vi "Read Single.vi"() -> ()   [LabVIEW 2013]
doc: "This example shows how to configure a measurement and take a reading."
uses:
  <instrlib>/Keithley 24XX/Public/Data/Read (Single Point).vi
  <vilib>/Utility/file.llb/Read From Spreadsheet File (DBL).vi
  <instrlib>/Keithley 24XX/Keithley 24XX.lvlib
  <vilib>/gmath/NI_Gmath.lvlib
panel:
  out "Temperature":dbl
  in  "定标文件":string(combo)
  in  "Source Mode  (0: Voltage)":u16(ring) items=["Voltage", "Current"]
  in  "Compliance  Level (0.1)":dbl=0.1
  in  "Output Level (0)":dbl
  in  "Enable Resistance Auto Range (T:Enable)":bool=TRUE
  in  "Enable Current Auto Range (T:Enable)":bool=TRUE
  in  "Enable Voltage Auto Range (T:Enable)":bool=TRUE
  in  "Resistance Manual Range (1.0)":dbl=1.0
  in  "Current Manual Range (1.0)":dbl=1.0
  in  "Voltage Manual Range (1.0)":dbl=1.0
  out "Resistance":sgl
  out "Current":sgl
  out "Voltage":sgl
  in  "Serial Configuration":T1={"Baud Rate"=9600, "Parity"=0, "Data Bits"=8, "Stop Bits"=10, "Flow Control"=0} {"Flow Control" items=["None", "XON/XOFF", "RTS/CTS", "XON/XOFF & RTS/CTS", "DTR/DSR", "XON/XOFF & DTR/DSR"]; "Stop Bits" items=["1.0"=10, "1.5"=15, "2.0"=20]; "Data Bits" items=["7"=7, "8"=8]; "Parity" items=["None", "Odd", "Even", "Mark", "Space"]; "Baud Rate" items=["300"=300, "600"=600, "1200"=1200, "2400"=2400, "4800"=4800, "9600"=9600, "19200"=19200]}
  in  "VISA resource name":refnum<visa-resource-name>
  # "Voltage Range Settings"
  # "Current Range Settings"
  # "Resistance Range Settings"
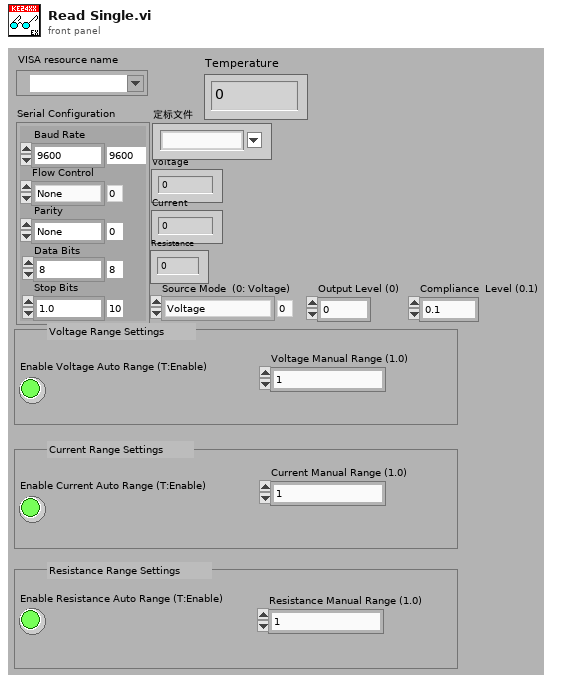
[diagram p1: front panel]
types:
  T1 = cluster{"Baud Rate":u32, "Parity":u16, "Data Bits":u16, "Stop Bits":u16, "Flow Control":u16}
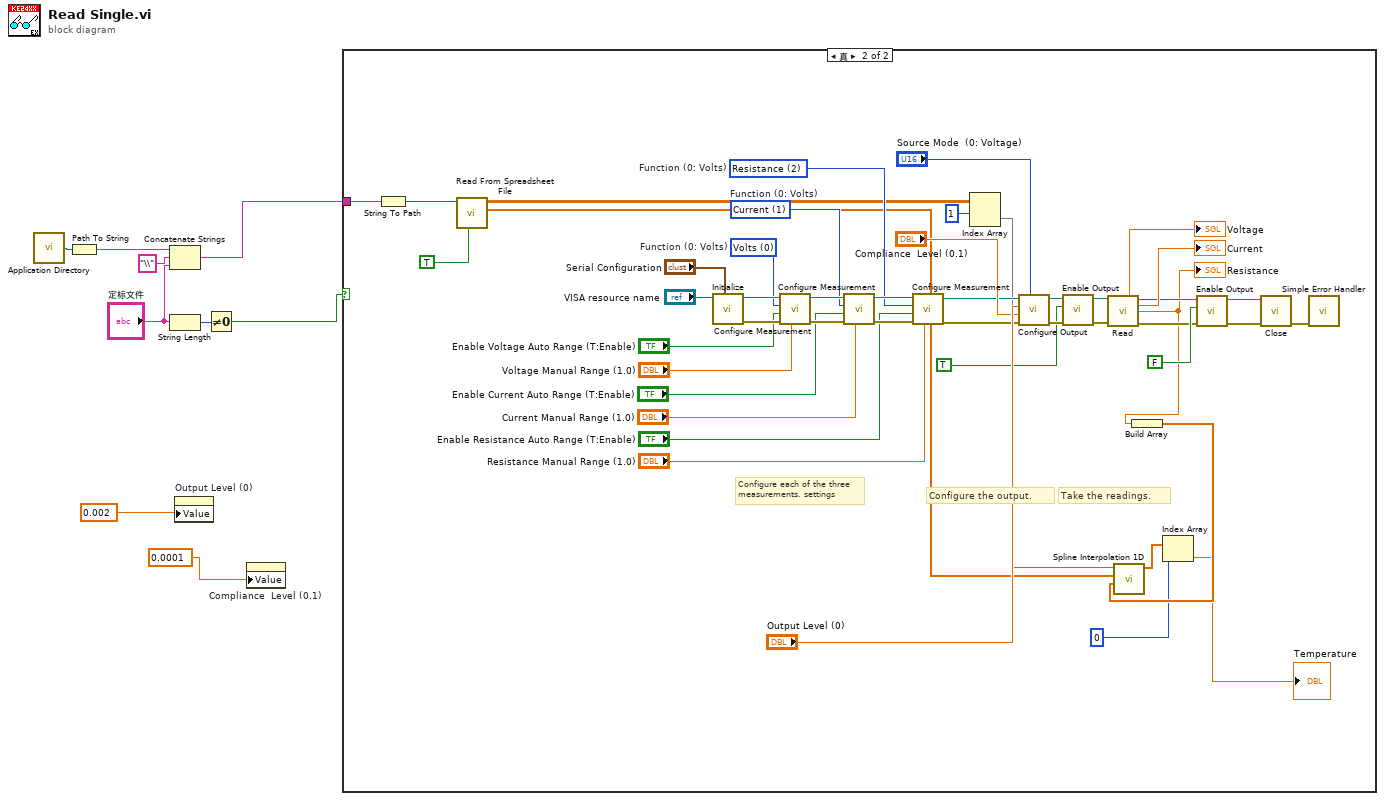
[diagram p0: block diagram]
diagram:
  n1 = call <vilib>:"Application Directory.vi"() -> ("Application Directory"=w9:path)
  n2 = Path To String(path=w9) -> (string=w8:string)
  n3 = Concatenate Strings(w8, "\\", "定标文件") -> (w3:string)
  n4 = String Length(string="定标文件") -> (length=w5:i32)
  n5 = property on="Output Level (0)" class="DigNum (严格)"("Value"=0.002) -> ()  [unwired: 2 in, 2 out]
  n6 = Not Equal To 0?(x=w5) -> (x != 0?=w4:bool)
  n7 = property on="Compliance  Level (0.1)" class="DigNum (严格)"("Value"=0.0001) -> ()  [unwired: 2 in, 2 out]
  n8 = case shown="真" w4 {
    tunnel: w3 -> [_ w16]
    frame False {
    }
    frame True {
      w43 = u16 2 items=["Volts", "Current", "Resistance"]  # Function (0: Volts)
      w44 = u16 1 items=["Volts", "Current", "Resistance"]  # Function (0: Volts)
      w45 = u16 0 items=["Volts", "Current", "Resistance"]  # Function (0: Volts)
      # "Take the readings."
      # "Configure the output."
      # "Configure each of the three measurements. settings"
      n9 = String To Path(string=w16) -> (path=w21:path)
      n10 = call-poly <vilib>:"Read From Spreadsheet File.vi"("transpose (no:F)"=TRUE, "file path (dialog if empty)"=w21) -> ("first row"=w18:dbl[], "all rows"=w19:dbl[][])  [unwired: 5 in, 3 out]
      n11 = call <instrlib>:"Initialize.vi"("Serial Configuration"="Serial Configuration", "VISA resource name"="VISA resource name") -> ("error out"=w50:errorcluster, "VISA resource name out"=w51:refnum<visa-resource-name>)  [unwired: 8 in]
      n12 = call <instrlib>:"Configure Measurement.vi"("Manual Range (1.0)"="Voltage Manual Range (1.0)", "error in (no error)"=w50, "Enable Auto Range (T:Enable)"="Enable Voltage Auto Range (T:Enable)", "Function (0: Volts)"=w45, "VISA resource name"=w51) -> ("error out"=w48:errorcluster, "VISA resource name out"=w49:refnum<visa-resource-name>)  [unwired: 5 in]
      n13 = call <instrlib>:"Configure Measurement.vi"("Manual Range (1.0)"="Current Manual Range (1.0)", "error in (no error)"=w48, "Enable Auto Range (T:Enable)"="Enable Current Auto Range (T:Enable)", "Function (0: Volts)"=w44, "VISA resource name"=w49) -> ("error out"=w47:errorcluster, "VISA resource name out"=w46:refnum<visa-resource-name>)  [unwired: 5 in]
      n14 = call <instrlib>:"Configure Measurement.vi"("Manual Range (1.0)"="Resistance Manual Range (1.0)", "error in (no error)"=w47, "Enable Auto Range (T:Enable)"="Enable Resistance Auto Range (T:Enable)", "Function (0: Volts)"=w43, "VISA resource name"=w46) -> ("error out"=w24:errorcluster, "VISA resource name out"=w23:refnum<visa-resource-name>)  [unwired: 5 in]
      n15 = Index Array(array=w19, index (row)=1) -> (element=w17:dbl[])  [unwired: 1 in]
      n16 = call <instrlib>:"Configure Output.vi"("Source Mode  (0: Voltage)"="Source Mode  (0: Voltage)", "error in (no error)"=w24, "Compliance  Level (0.1)"="Compliance  Level (0.1)", "Output Level (0)"="Output Level (0)", "VISA resource name"=w23) -> ("error out"=w26:errorcluster, "VISA resource name out"=w27:refnum<visa-resource-name>)  [unwired: 5 in]
      n17 = call <instrlib>:"Enable Output.vi"("error in (no error)"=w26, "Enable Output (T: Enable)"=TRUE, "VISA resource name"=w27) -> ("error out"=w29:errorcluster, "VISA resource name out"=w28:refnum<visa-resource-name>)  [unwired: 7 in]
      n18 = call-poly <instrlib>:"Read.vi"("VISA resource name"=w28, "error in (no error)"=w29) -> ("Voltage"=→"Voltage":sgl, "VISA resource name out"=w30:refnum<visa-resource-name>, "Current"=→"Current":sgl, "Resistance"=w15:sgl, "error out"=w31:errorcluster)  [unwired: 7 in, 2 out]
      "Resistance" <- w15
      n19 = Build Array(w15) -> (w14:sgl[])
      n20 = call <vilib>:"Spline Interpolation 1D.vi"("xi"=w14, "X"=w18, "Y"=w17) -> ("yi"=w13:dbl[])  [unwired: 6 in, 2 out]
      n21 = Index Array(array=w13, index=0) -> (element=→"Temperature":dbl)
      n22 = call <instrlib>:"Enable Output.vi"("error in (no error)"=w31, "Enable Output (T: Enable)"=FALSE, "VISA resource name"=w30) -> ("error out"=w32:errorcluster, "VISA resource name out"=w33:refnum<visa-resource-name>)  [unwired: 7 in]
      n23 = call <instrlib>:"Close.vi"("error in (no error)"=w32, "VISA resource name"=w33) -> ("error out"=w56:errorcluster)  [unwired: 9 in]
      n24 = call <vilib>:"Simple Error Handler.vi"("error in (no error)"=w56) -> ()  [unwired: 4 in, 5 out]
    }
  }
